vi "CMC_Homework06_Sub.vi"(2 "Grades":string[][](array[string]), 3 "Grade Cutoffs":T1, 4 "Use Grade Distrib":bool, 5 "error in (no error)":errorcluster) -> (0 "String":string, 1 "error out":errorcluster)   [LabVIEW 2013]
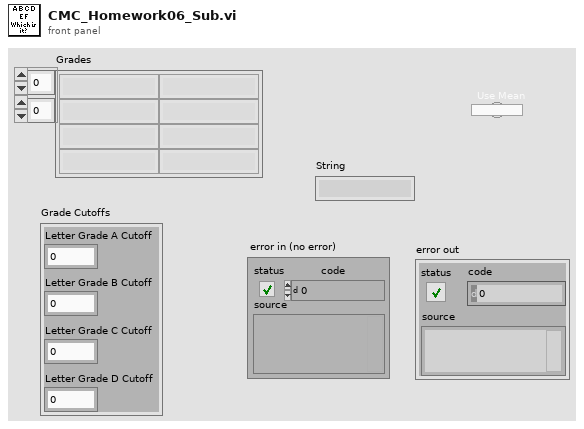
[diagram p1: front panel]
types:
  T1 = cluster{"Letter Grade D Cutoff":dbl, "Letter Grade C Cutoff":dbl, "Letter Grade B Cutoff":dbl, "Letter Grade A Cutoff":dbl}
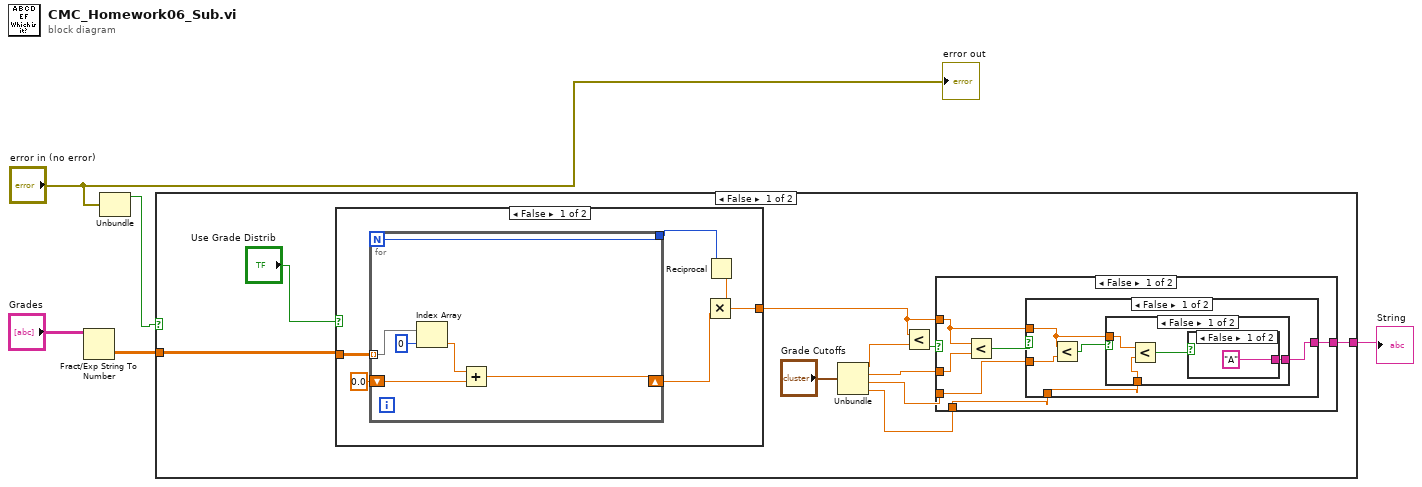
[diagram p0: block diagram]
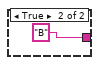
[diagram p2: hidden frame]
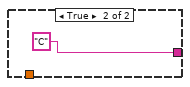
[diagram p3: hidden frame]
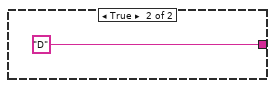
[diagram p4: hidden frame]
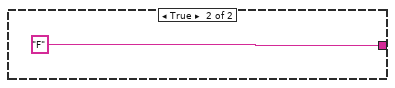
[diagram p5: hidden frame]
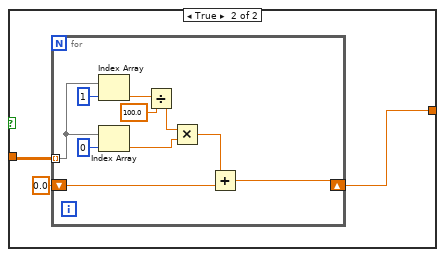
[diagram p6: hidden frame]
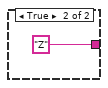
[diagram p7: hidden frame]
diagram:
  n1 = Fract/Exp String To Number(string="Grades") -> (number=w1:dbl[][])  [unwired: 3 in, 1 out]
  n2 = Unbundle("error in (no error)") -> ("status"=w3:bool)  [unwired: 2 out]
  n3 = case shown="False" w3 {
    tunnel: [w8 "Z"] -> w5
    tunnel: w1 -> [w6 _]
    frame False {
      n4 = case shown="False" "Use Grade Distrib" {
        tunnel: w6 -> [w41 w49]
        tunnel: [w37 w48] -> w9
        frame False {
          n5 = for {
            N -> [w42]
            tunnel: w41 -> [w47] mode=indexing
            shift-right: [w43] -> w39
            shift-left: 0.0 -> [w44]
            tunnel: [w42] -> w36
            n6 = Index Array(array=w47, index=0) -> (element=w45:dbl)
            n7 = Add(x=w45, y=w44) -> (x+y=w43:dbl)
          }
          n8 = Reciprocal(x=w36) -> (1/x=w38:dbl)
          n9 = Multiply(x=w38, y=w39) -> (x*y=w37:dbl)
        }
        frame True {
          n10 = for {
            tunnel: w49 -> [w58] mode=indexing
            shift-right: [w52] -> w48
            shift-left: 0.0 -> [w51]
            n11 = Index Array(array=w58, index=1) -> (element=w57:dbl)
            n12 = Index Array(array=w58, index=0) -> (element=w53:dbl)
            n13 = Divide(x=w57, y=100.0) -> (x/y=w54:dbl)
            n14 = Multiply(x=w54, y=w53) -> (x*y=w55:dbl)
            n15 = Add(x=w55, y=w51) -> (x+y=w52:dbl)
          }
        }
      }
      n16 = Unbundle("Grade Cutoffs") -> ("Letter Grade D Cutoff"=w14:dbl, "Letter Grade C Cutoff"=w12:dbl, "Letter Grade B Cutoff"=w11:dbl, "Letter Grade A Cutoff"=w10:dbl)
      n17 = Less?(x=w9, y=w14) -> (x < y?=w13:bool)
      n18 = case shown="False" w13 {
        tunnel: w12 -> [w21 _]
        tunnel: w11 -> [w17 _]
        tunnel: w10 -> [w16 _]
        tunnel: w9 -> [w19 _]
        tunnel: [w18 "F"] -> w8
        frame False {
          n19 = Less?(x=w19, y=w21) -> (x < y?=w20:bool)
          n20 = case shown="False" w20 {
            tunnel: w19 -> [w22 _]
            tunnel: [w23 "D"] -> w18
            tunnel: w17 -> [w25 _]
            tunnel: w16 -> [w24 _]
            frame False {
              n21 = Less?(x=w22, y=w25) -> (x < y?=w26:bool)
              n22 = case shown="False" w26 {
                tunnel: w24 -> [w30 _]
                tunnel: [w29 "C"] -> w23
                tunnel: w22 -> [w28 _]
                frame False {
                  n23 = Less?(x=w28, y=w30) -> (x < y?=w27:bool)
                  n24 = case shown="False" w27 {
                    tunnel: ["A" "B"] -> w29
                    frame False {
                    }
                    frame True {
                    }
                  }
                }
                frame True {
                }
              }
            }
            frame True {
            }
          }
        }
        frame True {
        }
      }
    }
    frame True {
    }
  }
  "String" <- w5
  "error out" <- "error in (no error)"
